vi "S4GUI.vi"(7 "Tab ObsEng":enum32{"Obs", "CCD modes", "Guider", "Eng"}(tab)) -> ()   [LabVIEW 2018] (continued)
        n2655 = call "Write ASEL.vi"("error in (no error)"=w5580, "Opt_Selector.lvclass"=w5582, "Instrument in"=w5591) -> ("error out"=w5542:errorcluster, "Instrument out"=w5558:refnum<class "Instrument.lvclass">)  [unwired: 7 in]
        n2656 = call "Read CALW.vi"("error in (no error)"=w5542, "Instrument in"=w5558) -> ("error out"=w5575:errorcluster, "Opt_Selector.lvclass"=w5576:refnum<class "Opt_Selector.lvclass">, "Instrument out"=w5557:refnum<class "Instrument.lvclass">)  [unwired: 7 in]
        n2657 = call-dynamic "Read State Machine.vi"("error in (no error)"=w5575, "Device in"=w5576) -> ("error out"=w5572:errorcluster, "State Machine.lvclass"=w5570:refnum<class "State Machine.lvclass">, "Device out"=w5578:refnum<class "Opt_Selector.lvclass">)  [unwired: 7 in]
        n2658 = call "Next State.vi"("error in (no error)"=w5572, "New_State"=1, "State Machine in"=w5570) -> ("error out"=w5573:errorcluster, "State Machine out"=w5574:refnum<class "State Machine.lvclass">)  [unwired: 7 in]
        n2659 = call-dynamic "Write State Machine.vi"("error in (no error)"=w5573, "State Machine.lvclass"=w5574, "Device in"=w5578) -> ("error out"=w5579:errorcluster, "Device out"=w5577:refnum<class "Opt_Selector.lvclass">)  [unwired: 7 in]
        n2660 = call "Write CALW.vi"("error in (no error)"=w5579, "Opt_Selector.lvclass"=w5577, "Instrument in"=w5557) -> ("error out"=w5541:errorcluster, "Instrument out"=w5556:refnum<class "Instrument.lvclass">)  [unwired: 7 in]
        n2661 = call "Read WPSEL.vi"("error in (no error)"=w5541, "Instrument in"=w5556) -> ("error out"=w5564:errorcluster, "Opt_Selector.lvclass"=w5563:refnum<class "Opt_Selector.lvclass">, "Instrument out"=w5555:refnum<class "Instrument.lvclass">)  [unwired: 7 in]
        n2662 = call-dynamic "Read State Machine.vi"("error in (no error)"=w5564, "Device in"=w5563) -> ("error out"=w5567:errorcluster, "State Machine.lvclass"=w5569:refnum<class "State Machine.lvclass">, "Device out"=w5561:refnum<class "Opt_Selector.lvclass">)  [unwired: 7 in]
        n2663 = call "Next State.vi"("error in (no error)"=w5567, "New_State"=1, "State Machine in"=w5569) -> ("error out"=w5566:errorcluster, "State Machine out"=w5565:refnum<class "State Machine.lvclass">)  [unwired: 7 in]
        n2664 = call-dynamic "Write State Machine.vi"("error in (no error)"=w5566, "State Machine.lvclass"=w5565, "Device in"=w5561) -> ("error out"=w5560:errorcluster, "Device out"=w5562:refnum<class "Opt_Selector.lvclass">)  [unwired: 7 in]
        n2665 = call "Write WPSEL.vi"("error in (no error)"=w5560, "Opt_Selector.lvclass"=w5562, "Instrument in"=w5555) -> ("error out"=w5540:errorcluster, "Instrument out"=w5544:refnum<class "Instrument.lvclass">)  [unwired: 7 in]
        n2666 = call "Read WPROT.vi"("error in (no error)"=w5540, "Instrument in"=w5544) -> ("error out"=w5550:errorcluster, "Opt_Selector.lvclass"=w5551:refnum<class "Opt_Selector.lvclass">, "Instrument out"=w5543:refnum<class "Instrument.lvclass">)  [unwired: 7 in]
        n2667 = call-dynamic "Read State Machine.vi"("error in (no error)"=w5550, "Device in"=w5551) -> ("error out"=w5547:errorcluster, "State Machine.lvclass"=w5545:refnum<class "State Machine.lvclass">, "Device out"=w5553:refnum<class "Opt_Selector.lvclass">)  [unwired: 7 in]
        n2668 = call "Next State.vi"("error in (no error)"=w5547, "New_State"=1, "State Machine in"=w5545) -> ("error out"=w5548:errorcluster, "State Machine out"=w5549:refnum<class "State Machine.lvclass">)  [unwired: 7 in]
        n2669 = call-dynamic "Write State Machine.vi"("error in (no error)"=w5548, "State Machine.lvclass"=w5549, "Device in"=w5553) -> ("error out"=w5554:errorcluster, "Device out"=w5552:refnum<class "Opt_Selector.lvclass">)  [unwired: 7 in]
        n2670 = call "Write WPROT.vi"("error in (no error)"=w5554, "Opt_Selector.lvclass"=w5552, "Instrument in"=w5543) -> ("error out"=w5516:errorcluster, "Instrument out"=w5517:refnum<class "Instrument.lvclass">)  [unwired: 7 in]
        n2671 = call "Read GMIR.vi"("error in (no error)"=w5516, "Instrument in"=w5517) -> ("error out"=w5535:errorcluster, "Opt_Continuous.lvclass"=w5536:refnum<class "Opt_Continuous.lvclass">, "Instrument out"=w5529:refnum<class "Instrument.lvclass">)  [unwired: 7 in]
        n2672 = call-dynamic "Read State Machine.vi"("error in (no error)"=w5535, "Device in"=w5536) -> ("error out"=w5532:errorcluster, "State Machine.lvclass"=w5530:refnum<class "State Machine.lvclass">, "Device out"=w5538:refnum<class "Opt_Continuous.lvclass">)  [unwired: 7 in]
        n2673 = call "Next State.vi"("error in (no error)"=w5532, "New_State"=1, "State Machine in"=w5530) -> ("error out"=w5533:errorcluster, "State Machine out"=w5534:refnum<class "State Machine.lvclass">)  [unwired: 7 in]
        n2674 = call-dynamic "Write State Machine.vi"("error in (no error)"=w5533, "State Machine.lvclass"=w5534, "Device in"=w5538) -> ("error out"=w5539:errorcluster, "Device out"=w5537:refnum<class "Opt_Continuous.lvclass">)  [unwired: 7 in]
        n2675 = call "Write GMIR.vi"("error in (no error)"=w5539, "Opt_Continuous.lvclass"=w5537, "Instrument in"=w5529) -> ("error out"=w5514:errorcluster, "Instrument out"=w5515:refnum<class "Instrument.lvclass">)  [unwired: 7 in]
        n2676 = call "Read GFOC.vi"("error in (no error)"=w5514, "Instrument in"=w5515) -> ("error out"=w5524:errorcluster, "Opt_Continuous.lvclass"=w5525:refnum<class "Opt_Continuous.lvclass">, "Instrument out"=w5518:refnum<class "Instrument.lvclass">)  [unwired: 7 in]
        n2677 = call-dynamic "Read State Machine.vi"("error in (no error)"=w5524, "Device in"=w5525) -> ("error out"=w5521:errorcluster, "State Machine.lvclass"=w5519:refnum<class "State Machine.lvclass">, "Device out"=w5527:refnum<class "Opt_Continuous.lvclass">)  [unwired: 7 in]
        n2678 = call "Next State.vi"("error in (no error)"=w5521, "New_State"=1, "State Machine in"=w5519) -> ("error out"=w5522:errorcluster, "State Machine out"=w5523:refnum<class "State Machine.lvclass">)  [unwired: 7 in]
        n2679 = call-dynamic "Write State Machine.vi"("error in (no error)"=w5522, "State Machine.lvclass"=w5523, "Device in"=w5527) -> ("error out"=w5528:errorcluster, "Device out"=w5526:refnum<class "Opt_Continuous.lvclass">)  [unwired: 7 in]
        n2680 = call "Write GFOC.vi"("error in (no error)"=w5528, "Opt_Continuous.lvclass"=w5526, "Instrument in"=w5518) -> ("error out"=w5510:errorcluster, "Instrument out"=w5511:refnum<class "Instrument.lvclass">)  [unwired: 7 in]
        n2681 = call "Write Instrument.lvclass.vi"("error in (no error)"=w5510, "Instrument.lvclass"=w5511, "S4ACS_GUI in"=w5590) -> ("error out"=w5509:errorcluster, "S4ACS_GUI out"=w5508:refnum<class "S4GUI.lvclass">)  [unwired: 7 in]
      }
      event "Tab Acq Type": Value Change {
        # "Tab for choosing ACQUISITION MODE: Object, Test, Dflat, Sflat, Dark, Zero, Focus"
        n2682 = event-data() -> ("NewVal"=w5631:T1)  [unwired: 1 in]
        n2683 = case shown="\"TEST\"" w5631 {
          tunnel: ["OBJECT" "OBJECT" "FLAT" "FLAT" "DARK" "ZERO" "FOCUS"] -> w5608
          tunnel: [w5700 w5705 w5713 w5718 w5723 w5728 w5733] -> w5607
          tunnel: [w5701 w5706 w5712 w5717 w5722 w5727 w5732] -> w5630
          tunnel: [w5702 w5707 w5711 w5716 w5721 w5726 w5731] -> w5604
          tunnel: [u32 0 u32 1 u32 2 u32 3 u32 4 u32 5 u32 6] -> w5593
          frame "OBJECT", Default {
            n2684 = local read "Object_obj"() -> (w5700:string)
            n2685 = local read "OBJECT Comments"() -> (w5702:string)
            n2686 = local read "object suffix"() -> (w5701:string)
          }
          frame "TEST" {
            n2687 = local read "TEST Comments"() -> (w5707:string)
            n2688 = local read "Object_test"() -> (w5705:string)
            n2689 = local read "test suffix"() -> (w5706:string)
          }
          frame "DFLAT" {
            n2690 = local read "DFLAT Comments"() -> (w5711:string)
            n2691 = local read "Object_dflat"() -> (w5713:string)
            n2692 = local read "dflat suffix"() -> (w5712:string)
          }
          frame "SFLAT" {
            n2693 = local read "SFLAT Comments"() -> (w5716:string)
            n2694 = local read "Object_sflat"() -> (w5718:string)
            n2695 = local read "sflat suffix"() -> (w5717:string)
          }
          frame "DARK" {
            n2696 = local read "Object_dark"() -> (w5723:string)
            n2697 = local read "dark suffix"() -> (w5722:string)
            n2698 = local read "DARK Comments"() -> (w5721:string)
          }
          frame "ZERO" {
            n2699 = local read "ZERO Comments"() -> (w5726:string)
            n2700 = local read "Object_zero"() -> (w5728:string)
            n2701 = local read "zero suffix"() -> (w5727:string)
          }
          frame "FOCUS" {
            n2702 = local read "FOCUS Comments"() -> (w5731:string)
            n2703 = local read "Object_focus"() -> (w5733:string)
            n2704 = local read "focus suffix"() -> (w5732:string)
          }
        }
        n2705 = local read "Observer"() -> (w5629:string)
        n2706 = call-dynamic "Write ExpMode.vi"("error in (no error)"=w5632, "ExpMode"=w5631, "S4GUI in"=w5633) -> ("error out"=w5625:errorcluster, "S4GUI out"=w5624:refnum<class "S4GUI.lvclass">)  [unwired: 7 in]
        n2707 = Concatenate Strings("ACQ TAB SELECTED:" ("User Event"), w5608) -> (w5626:string)
        n2708 = call-dynamic "Write User Event.vi"("error in (no error)"=w5625, "User Event"=w5626, "S4GUI in"=w5624) -> ("error out"=w5598:errorcluster, "S4GUI out"=w5599:refnum<class "S4GUI.lvclass">)  [unwired: 7 in]
        n2709 = call-dynamic "Write TabAcqType index.vi"("error in (no error)"=w5598, "TabAcqType index"=w5593, "S4GUI in"=w5599) -> ("error out"=w5597:errorcluster, "S4GUI out"=w5595:refnum<class "S4GUI.lvclass">)  [unwired: 7 in]
        n2710 = call-dynamic "Save TabAcqType index.vi"("error in (no error)"=w5597, "S4GUI in"=w5595) -> ("error out"=w5596:errorcluster, "S4GUI out"=w5594:refnum<class "S4GUI.lvclass">)  [unwired: 8 in]
        n2711 = call-dynamic "Read Publisher.lvclass.vi"("error in (no error)"=w5596, "S4GUI in"=w5594) -> ("error out"=w5622:errorcluster, "Publisher.lvclass"=w5618:refnum<class "Publisher.lvclass">, "S4GUI out"=w5623:refnum<class "S4GUI.lvclass">)  [unwired: 7 in]
        n2712 = call-dynamic "Write object.vi"("error in (no error)"=w5622, "object"=w5607, "Publisher in"=w5618) -> ("error out"=w5621:errorcluster, "Publisher out"=w5617:refnum<class "Publisher.lvclass">)  [unwired: 7 in]
        n2713 = call-dynamic "Write obstype.vi"("error in (no error)"=w5621, "obstype"=w5608, "Publisher in"=w5617) -> ("error out"=w5620:errorcluster, "Publisher out"=w5616:refnum<class "Publisher.lvclass">)  [unwired: 7 in]
        n2714 = call-dynamic "Write observer.vi"("error in (no error)"=w5620, "observer"=w5606, "Publisher in"=w5616) -> ("error out"=w5619:errorcluster, "Publisher out"=w5615:refnum<class "Publisher.lvclass">)  [unwired: 7 in]
        n2715 = call-dynamic "Write projid.vi"("error in (no error)"=w5619, "projid"=w5605, "Publisher in"=w5615) -> ("error out"=w5612:errorcluster, "Publisher out"=w5611:refnum<class "Publisher.lvclass">)  [unwired: 7 in]
        n2716 = call-dynamic "Write comments.vi"("error in (no error)"=w5612, "comments"=w5604, "Publisher in"=w5611) -> ("error out"=w5614:errorcluster, "Publisher out"=w5613:refnum<class "Publisher.lvclass">)  [unwired: 7 in]
        n2717 = call-dynamic "Write Publisher.lvclass.vi"("error in (no error)"=w5614, "Publisher.lvclass"=w5613, "S4GUI in"=w5623) -> ("error out"=w5610:errorcluster, "S4GUI out"=w5609:refnum<class "S4GUI.lvclass">)  [unwired: 7 in]
        n2718 = call-dynamic "Read AcquisitionA.vi"("error in (no error)"=w5610, "S4ACS_GUI in"=w5609) -> ("error out"=w5640:errorcluster, "Acquisition.lvclass"=w5641:refnum<class "Acquisition.lvclass">, "S4ACS_GUI out"=w5660:refnum<class "S4GUI.lvclass">)  [unwired: 7 in]
        n2719 = call-dynamic "Read AcquisitionC.vi"("error in (no error)"=w5596, "S4ACS_GUI in"=w5594) -> ("error out"=w5636:errorcluster, "Acquisition.lvclass"=w5637:refnum<class "Acquisition.lvclass">)  [unwired: 7 in, 1 out]
        n2720 = call "Read AcquisitionB.vi"("error in (no error)"=w5596, "S4ACS_GUI in"=w5594) -> ("error out"=w5638:errorcluster, "Acquisition.lvclass"=w5639:refnum<class "Acquisition.lvclass">)  [unwired: 7 in, 1 out]
        n2721 = call-dynamic "Read AcquisitionD.vi"("error in (no error)"=w5596, "S4ACS_GUI in"=w5594) -> ("error out"=w5634:errorcluster, "Acquisition.lvclass"=w5635:refnum<class "Acquisition.lvclass">)  [unwired: 7 in, 1 out]
        n2722 = To Lower Case(string=w5630) -> (all lower case string=w5628:string)
        n2723 = case shown="\"OBJECT\", Default" w5631 {
          tunnel: [w5968 w6337 w6770] -> w5659
          tunnel: [w5967 w6336 w6769] -> w5658
          tunnel: [w5966 w6335 w6768] -> w5656
          tunnel: [w5965 w6334 w6767] -> w5655
          tunnel: [w5964 w6333 w6766] -> w5645
          tunnel: [w5963 w6332 w6765] -> w5644
          tunnel: [w5962 w6331 w6764] -> w5643
          tunnel: [w5961 w6330 w6763] -> w5642
          tunnel: w5641 -> [w5960 w6329 w6762]
          tunnel: w5640 -> [w5959 w6328 w6761]
          tunnel: w5639 -> [w5949 w6319 w6752]
          tunnel: w5638 -> [w5948 w6318 w6751]
          tunnel: w5637 -> [w5947 w6317 w6750]
          tunnel: w5636 -> [w5946 w6316 w6749]
          tunnel: w5635 -> [w5945 w6315 w6748]
          tunnel: w5634 -> [w5944 w6314 w6747]
          tunnel: w5607 -> [w5941 w6313 w6746]
          tunnel: w5604 -> [w5942 w6312 w6745]
          tunnel: w5629 -> [w5943 w6311 w6744]
          tunnel: w5628 -> [w5940 w6310 w6743]
          tunnel: w5608 -> [w5939 w6309 w6742]
          frame "ZERO" {
            w5958 = 1e-05 ("Exptime ch1")
            # "nome do arquivo .cfg"
            # "seção no arquivo .cfg"
            # "nome do arquivo .cfg"
            # "seção no arquivo .cfg"
            # "nome do arquivo .cfg"
            # "seção no arquivo .cfg"
            # "nome do arquivo .cfg"
            # "seção no arquivo .cfg"
            # "ZERO: EXPTIME=1E-5 (mandatory), shutter automatically closed, save current FRAME_TRANSFER (prev_FT) and reset FRAME_TRANSFER."
            n2724 = call "Read connection.vi"("error in (no error)"=w5946, "Server in"=w5947) -> ("error out"=w5952:errorcluster, "connection"=w5786:bool, "Server out"=w5953:refnum<class "Acquisition.lvclass">)  [unwired: 7 in]
            n2725 = call "Read connection.vi"("error in (no error)"=w5948, "Server in"=w5949) -> ("error out"=w5954:errorcluster, "connection"=w5837:bool, "Server out"=w5955:refnum<class "Acquisition.lvclass">)  [unwired: 7 in]
            n2726 = call "Read connection.vi"("error in (no error)"=w5959, "Server in"=w5960) -> ("error out"=w5956:errorcluster, "connection"=w5888:bool, "Server out"=w5957:refnum<class "Acquisition.lvclass">)  [unwired: 7 in]
            n2727 = call "Read connection.vi"("error in (no error)"=w5944, "Server in"=w5945) -> ("error out"=w5950:errorcluster, "connection"=w5735:bool, "Server out"=w5951:refnum<class "Acquisition.lvclass">)  [unwired: 7 in]
            n2728 = call-dynamic "Read Channel.vi"("error in (no error)"=w5954, "Acquisition in"=w5955) -> ("error out"=w5875:errorcluster, "Channel.lvclass"=w5874:refnum<class "Channel.lvclass">, "Acquisition out"=w5873:refnum<class "Acquisition.lvclass">)  [unwired: 7 in]
            n2729 = call-dynamic "Read Channel.vi"("error in (no error)"=w5950, "Acquisition in"=w5951) -> ("error out"=w5783:errorcluster, "Channel.lvclass"=w5784:refnum<class "Channel.lvclass">, "Acquisition out"=w5785:refnum<class "Acquisition.lvclass">)  [unwired: 7 in]
            n2730 = call-dynamic "Read Channel.vi"("error in (no error)"=w5952, "Acquisition in"=w5953) -> ("error out"=w5824:errorcluster, "Channel.lvclass"=w5823:refnum<class "Channel.lvclass">, "Acquisition out"=w5822:refnum<class "Acquisition.lvclass">)  [unwired: 7 in]
            n2731 = call-dynamic "Read Channel.vi"("error in (no error)"=w5956, "Acquisition in"=w5957) -> ("error out"=w5936:errorcluster, "Channel.lvclass"=w5937:refnum<class "Channel.lvclass">, "Acquisition out"=w5938:refnum<class "Acquisition.lvclass">)  [unwired: 7 in]
            n2732 = call-dynamic "Read Interface.vi"("error in (no error)"=w5783, "Channel in"=w5784) -> ("error out"=w5749:errorcluster, "Interface.lvclass"=w5748:refnum<class "Interface.lvclass">, "Channel out"=w5745:refnum<class "Channel.lvclass">)  [unwired: 7 in]
            n2733 = call-dynamic "Read Interface.vi"("error in (no error)"=w5875, "Channel in"=w5874) -> ("error out"=w5849:errorcluster, "Interface.lvclass"=w5850:refnum<class "Interface.lvclass">, "Channel out"=w5844:refnum<class "Channel.lvclass">)  [unwired: 7 in]
            n2734 = call-dynamic "Read Interface.vi"("error in (no error)"=w5824, "Channel in"=w5823) -> ("error out"=w5798:errorcluster, "Interface.lvclass"=w5799:refnum<class "Interface.lvclass">, "Channel out"=w5796:refnum<class "Channel.lvclass">)  [unwired: 7 in]
            n2735 = call-dynamic "Read Interface.vi"("error in (no error)"=w5936, "Channel in"=w5937) -> ("error out"=w5905:errorcluster, "Interface.lvclass"=w5906:refnum<class "Interface.lvclass">, "Channel out"=w5899:refnum<class "Channel.lvclass">)  [unwired: 7 in]
            n2736 = call-dynamic "Write restoreExpTime.vi"("error in (no error)"=w5749, "restoreExpTime"=TRUE, "Interface in"=w5748) -> ("error out"=w5742:errorcluster, "Interface out"=w5747:refnum<class "Interface.lvclass">)  [unwired: 7 in]
            n2737 = call-dynamic "Write restoreExpTime.vi"("error in (no error)"=w5849, "restoreExpTime"=TRUE, "Interface in"=w5850) -> ("error out"=w5846:errorcluster, "Interface out"=w5848:refnum<class "Interface.lvclass">)  [unwired: 7 in]
            n2738 = call-dynamic "Write restoreExpTime.vi"("error in (no error)"=w5798, "restoreExpTime"=TRUE, "Interface in"=w5799) -> ("error out"=w5791:errorcluster, "Interface out"=w5797:refnum<class "Interface.lvclass">)  [unwired: 7 in]
            n2739 = call-dynamic "Write restoreExpTime.vi"("error in (no error)"=w5905, "restoreExpTime"=TRUE, "Interface in"=w5906) -> ("error out"=w5895:errorcluster, "Interface out"=w5896:refnum<class "Interface.lvclass">)  [unwired: 7 in]
            n2740 = property on="Exptime ch1" class="DigNum (strict)"("Value"=w5958) -> ()  [unwired: 2 in, 2 out]
            n2741 = call-dynamic "Read target cluster.vi"("error in (no error)"=w5846, "Channel in"=w5844) -> ("error out"=w5845:errorcluster, "target cluster"=w5847:T31, "Channel out"=w5840:refnum<class "Channel.lvclass">)  [unwired: 7 in]
            n2742 = stacked-sequence {
              tunnel: [_ w6060] -> w5843
              tunnel: w5847 -> [_ w6059]
              tunnel: w5847 -> [w6057 _]
              tunnel: [w6056 _] -> w5852
              frame #0 {
                n2743 = Unbundle By Name(w6057) -> ("FRAME_TRANSFER"=w6056:bool)
              }
              frame #1 {
                # "closed"
                n2744 = Bundle By Name(cluster=w6059, "SHUTTER_MODE"=u8 2, "FRAME_TRANSFER"=FALSE) -> (w6060:T31)
              }
            }
            n2745 = call-dynamic "Read target cluster.vi"("error in (no error)"=w5742, "Channel in"=w5745) -> ("error out"=w5741:errorcluster, "target cluster"=w5743:T31, "Channel out"=w5744:refnum<class "Channel.lvclass">)  [unwired: 7 in]
            n2746 = stacked-sequence {
              tunnel: w5743 -> [_ w5999]
              tunnel: [_ w5998] -> w5739
              tunnel: w5743 -> [w5995 _]
              tunnel: [w5994 _] -> w5751
              frame #0 {
                n2747 = Unbundle By Name(w5995) -> ("FRAME_TRANSFER"=w5994:bool)
              }
              frame #1 {
                # "closed"
                n2748 = Bundle By Name(cluster=w5999, "SHUTTER_MODE"=u8 2, "FRAME_TRANSFER"=FALSE) -> (w5998:T31)
              }
            }
            n2749 = call-dynamic "Read target cluster.vi"("error in (no error)"=w5791, "Channel in"=w5796) -> ("error out"=w5790:errorcluster, "target cluster"=w5792:T31, "Channel out"=w5788:refnum<class "Channel.lvclass">)  [unwired: 7 in]
            n2750 = stacked-sequence {
              tunnel: [_ w6029] -> w5794
              tunnel: w5792 -> [_ w6028]
              tunnel: w5792 -> [w6026 _]
              tunnel: [w6025 _] -> w5801
              frame #0 {
                n2751 = Unbundle By Name(w6026) -> ("FRAME_TRANSFER"=w6025:bool)
              }
              frame #1 {
                # "closed"
                n2752 = Bundle By Name(cluster=w6028, "SHUTTER_MODE"=u8 2, "FRAME_TRANSFER"=FALSE) -> (w6029:T31)
              }
            }
            n2753 = property on="Exptime ch2" class="DigNum (strict)"("Value"=w5958) -> ()  [unwired: 2 in, 2 out]
            n2754 = call-dynamic "Read target cluster.vi"("error in (no error)"=w5895, "Channel in"=w5899) -> ("error out"=w5894:errorcluster, "target cluster"=w5897:T31, "Channel out"=w5898:refnum<class "Channel.lvclass">)  [unwired: 7 in]
            n2755 = stacked-sequence {
              tunnel: [_ w6092] -> w5903
              tunnel: w5897 -> [_ w6089]
              tunnel: w5897 -> [w6088 _]
              tunnel: [w6087 _] -> w5907
              frame #0 {
                n2756 = Unbundle By Name(w6088) -> ("FRAME_TRANSFER"=w6087:bool)
              }
              frame #1 {
                # "closed"
                n2757 = Bundle By Name(cluster=w6089, "SHUTTER_MODE"=u8 2, "FRAME_TRANSFER"=FALSE) -> (w6092:T31)
              }
            }
            n2758 = call-dynamic "Write PREV_FT.vi"("error in (no error)"=w5845, "PREV_FT"=w5852, "Interface in"=w5848) -> ("error out"=w5842:errorcluster, "Interface out"=w5838:refnum<class "Interface.lvclass">)  [unwired: 7 in]
            n2759 = call-dynamic "Write PREV_FT.vi"("error in (no error)"=w5741, "PREV_FT"=w5751, "Interface in"=w5747) -> ("error out"=w5740:errorcluster, "Interface out"=w5746:refnum<class "Interface.lvclass">)  [unwired: 7 in]
            n2760 = call-dynamic "Write PREV_FT.vi"("error in (no error)"=w5790, "PREV_FT"=w5801, "Interface in"=w5797) -> ("error out"=w5793:errorcluster, "Interface out"=w5795:refnum<class "Interface.lvclass">)  [unwired: 7 in]
            n2761 = property on="Exptime ch3" class="DigNum (strict)"("Value"=w5958) -> ()  [unwired: 2 in, 2 out]
            n2762 = call-dynamic "Write PREV_FT.vi"("error in (no error)"=w5894, "PREV_FT"=w5907, "Interface in"=w5896) -> ("error out"=w5900:errorcluster, "Interface out"=w5893:refnum<class "Interface.lvclass">)  [unwired: 7 in]
            n2763 = call-dynamic "Write target cluster.vi"("error in (no error)"=w5842, "target cluster"=w5843, "Channel in"=w5840) -> ("error out"=w5841:errorcluster, "Channel out"=w5839:refnum<class "Channel.lvclass">)  [unwired: 7 in]
            n2764 = call-dynamic "Write target cluster.vi"("error in (no error)"=w5740, "target cluster"=w5739, "Channel in"=w5744) -> ("error out"=w5738:errorcluster, "Channel out"=w5737:refnum<class "Channel.lvclass">)  [unwired: 7 in]
            n2765 = call-dynamic "Write target cluster.vi"("error in (no error)"=w5793, "target cluster"=w5794, "Channel in"=w5788) -> ("error out"=w5789:errorcluster, "Channel out"=w5787:refnum<class "Channel.lvclass">)  [unwired: 7 in]
            n2766 = call-dynamic "Write target cluster.vi"("error in (no error)"=w5900, "target cluster"=w5903, "Channel in"=w5898) -> ("error out"=w5902:errorcluster, "Channel out"=w5901:refnum<class "Channel.lvclass">)  [unwired: 7 in]
            n2767 = Flatten To String(anything=w5843, error in (no error)=w5841) -> (data string=w5876:string, error out=w5877:errorcluster)  [unwired: 2 in, 1 out]
            n2768 = Flatten To String(anything=w5739, error in (no error)=w5738) -> (data string=w5782:string, error out=w5781:errorcluster)  [unwired: 2 in, 1 out]
            n2769 = Flatten To String(anything=w5794, error in (no error)=w5789) -> (data string=w5825:string, error out=w5826:errorcluster)  [unwired: 2 in, 1 out]
            n2770 = Flatten To String(anything=w5903, error in (no error)=w5902) -> (data string=w5935:string, error out=w5934:errorcluster)  [unwired: 2 in, 1 out]
            n2771 = property on="Exptime ch4" class="DigNum (strict)"("Value"=w5958) -> ()  [unwired: 2 in, 2 out]
            n2772 = call "Write flatted cluster.vi"("error in (no error)"=w5877, "flatted cluster"=w5876, "Interface in"=w5838) -> ("error out"=w5879:errorcluster, "Interface out"=w5878:refnum<class "Interface.lvclass">)  [unwired: 7 in]
            n2773 = call "Write flatted cluster.vi"("error in (no error)"=w5781, "flatted cluster"=w5782, "Interface in"=w5746) -> ("error out"=w5779:errorcluster, "Interface out"=w5780:refnum<class "Interface.lvclass">)  [unwired: 7 in]
            n2774 = call "Write flatted cluster.vi"("error in (no error)"=w5826, "flatted cluster"=w5825, "Interface in"=w5795) -> ("error out"=w5828:errorcluster, "Interface out"=w5827:refnum<class "Interface.lvclass">)  [unwired: 7 in]
            n2775 = call "Write flatted cluster.vi"("error in (no error)"=w5934, "flatted cluster"=w5935, "Interface in"=w5893) -> ("error out"=w5932:errorcluster, "Interface out"=w5933:refnum<class "Interface.lvclass">)  [unwired: 7 in]
            n2776 = call-dynamic "Write Interface.vi"("error in (no error)"=w5879, "Interface.lvclass"=w5878, "Channel in"=w5839) -> ("error out"=w5881:errorcluster, "Channel out"=w5882:refnum<class "Channel.lvclass">)  [unwired: 7 in]
            n2777 = call-dynamic "Write Interface.vi"("error in (no error)"=w5779, "Interface.lvclass"=w5780, "Channel in"=w5737) -> ("error out"=w5777:errorcluster, "Channel out"=w5776:refnum<class "Channel.lvclass">)  [unwired: 7 in]
            n2778 = call-dynamic "Write Interface.vi"("error in (no error)"=w5828, "Interface.lvclass"=w5827, "Channel in"=w5787) -> ("error out"=w5830:errorcluster, "Channel out"=w5831:refnum<class "Channel.lvclass">)  [unwired: 7 in]
            n2779 = call-dynamic "Write Interface.vi"("error in (no error)"=w5932, "Interface.lvclass"=w5933, "Channel in"=w5901) -> ("error out"=w5930:errorcluster, "Channel out"=w5929:refnum<class "Channel.lvclass">)  [unwired: 7 in]
            n2780 = call "Write section_name.vi"("error in (no error)"=w5881, "section_name"="CCD_ACS2", "Channel in"=w5882) -> ("error out"=w5880:errorcluster, "Channel out"=w5885:refnum<class "Channel.lvclass">)  [unwired: 7 in]
            n2781 = call "Write section_name.vi"("error in (no error)"=w5777, "section_name"="CCD_ACS4", "Channel in"=w5776) -> ("error out"=w5778:errorcluster, "Channel out"=w5773:refnum<class "Channel.lvclass">)  [unwired: 7 in]
            n2782 = call "Write section_name.vi"("error in (no error)"=w5830, "section_name"="CCD_ACS3", "Channel in"=w5831) -> ("error out"=w5829:errorcluster, "Channel out"=w5834:refnum<class "Channel.lvclass">)  [unwired: 7 in]
            n2783 = call "Write section_name.vi"("error in (no error)"=w5930, "section_name"="CCD_ACS1", "Channel in"=w5929) -> ("error out"=w5931:errorcluster, "Channel out"=w5926:refnum<class "Channel.lvclass">)  [unwired: 7 in]
            n2784 = call-dynamic "save config.vi"("error in (no error)"=w5880, "file config"="lastsaved.cfg", "Channel in"=w5885) -> ("error out"=w5855:errorcluster, "Channel out"=w5856:refnum<class "Channel.lvclass">)  [unwired: 7 in]
            n2785 = call-dynamic "save config.vi"("error in (no error)"=w5778, "file config"="lastsaved.cfg", "Channel in"=w5773) -> ("error out"=w5754:errorcluster, "Channel out"=w5755:refnum<class "Channel.lvclass">)  [unwired: 7 in]
            n2786 = call-dynamic "save config.vi"("error in (no error)"=w5829, "file config"="lastsaved.cfg", "Channel in"=w5834) -> ("error out"=w5803:errorcluster, "Channel out"=w5805:refnum<class "Channel.lvclass">)  [unwired: 7 in]
            n2787 = call-dynamic "save config.vi"("error in (no error)"=w5931, "file config"="lastsaved.cfg", "Channel in"=w5926) -> ("error out"=w5916:errorcluster, "Channel out"=w5917:refnum<class "Channel.lvclass">)  [unwired: 7 in]
            n2788 = local read "Filter2"() -> (w5857:u8)
            n2789 = local read "Filter4"() -> (w5771:u8)
            n2790 = local read "Filter3"() -> (w5821:u8)
            n2791 = local read "Filter1"() -> (w5918:u8)
            n2792 = call-dynamic "Write Filter.vi"("error in (no error)"=w5855, "Filter"=w5857, "Channel in"=w5856) -> ("error out"=w5864:errorcluster, "Channel out"=w5865:refnum<class "Channel.lvclass">)  [unwired: 7 in]
            n2793 = call-dynamic "Write Filter.vi"("error in (no error)"=w5754, "Filter"=w5771, "Channel in"=w5755) -> ("error out"=w5764:errorcluster, "Channel out"=w5763:refnum<class "Channel.lvclass">)  [unwired: 7 in]
            n2794 = call-dynamic "Write Filter.vi"("error in (no error)"=w5803, "Filter"=w5821, "Channel in"=w5805) -> ("error out"=w5814:errorcluster, "Channel out"=w5813:refnum<class "Channel.lvclass">)  [unwired: 7 in]
            n2795 = call-dynamic "Write Filter.vi"("error in (no error)"=w5916, "Filter"=w5918, "Channel in"=w5917) -> ("error out"=w5925:errorcluster, "Channel out"=w5915:refnum<class "Channel.lvclass">)  [unwired: 7 in]
            n2796 = call-dynamic "Read Interface.vi"("error in (no error)"=w5864, "Channel in"=w5865) -> ("error out"=w5862:errorcluster, "Interface.lvclass"=w5867:refnum<class "Interface.lvclass">, "Channel out"=w5866:refnum<class "Channel.lvclass">)  [unwired: 7 in]
            n2797 = call-dynamic "Read Interface.vi"("error in (no error)"=w5764, "Channel in"=w5763) -> ("error out"=w5766:errorcluster, "Interface.lvclass"=w5761:refnum<class "Interface.lvclass">, "Channel out"=w5762:refnum<class "Channel.lvclass">)  [unwired: 7 in]
            n2798 = call-dynamic "Read Interface.vi"("error in (no error)"=w5814, "Channel in"=w5813) -> ("error out"=w5816:errorcluster, "Interface.lvclass"=w5811:refnum<class "Interface.lvclass">, "Channel out"=w5812:refnum<class "Channel.lvclass">)  [unwired: 7 in]
            n2799 = call-dynamic "Read Interface.vi"("error in (no error)"=w5925, "Channel in"=w5915) -> ("error out"=w5923:errorcluster, "Interface.lvclass"=w5914:refnum<class "Interface.lvclass">, "Channel out"=w5908:refnum<class "Channel.lvclass">)  [unwired: 7 in]
            n2800 = call-dynamic "Write Suffix.vi"("error in (no error)"=w5862, "Suffix"=w5940, "Interface in"=w5867) -> ("error out"=w5858:errorcluster, "Interface out"=w5868:refnum<class "Interface.lvclass">)  [unwired: 7 in]
            n2801 = call-dynamic "Write Suffix.vi"("error in (no error)"=w5766, "Suffix"=w5940, "Interface in"=w5761) -> ("error out"=w5770:errorcluster, "Interface out"=w5760:refnum<class "Interface.lvclass">)  [unwired: 7 in]
            n2802 = call-dynamic "Write Suffix.vi"("error in (no error)"=w5816, "Suffix"=w5940, "Interface in"=w5811) -> ("error out"=w5820:errorcluster, "Interface out"=w5810:refnum<class "Interface.lvclass">)  [unwired: 7 in]
            n2803 = call-dynamic "Write Suffix.vi"("error in (no error)"=w5923, "Suffix"=w5940, "Interface in"=w5914) -> ("error out"=w5919:errorcluster, "Interface out"=w5913:refnum<class "Interface.lvclass">)  [unwired: 7 in]
            n2804 = call-dynamic "Write ObsType.vi"("error in (no error)"=w5858, "ObsType"=w5939, "Interface in"=w5868) -> ("error out"=w5859:errorcluster, "Interface out"=w5869:refnum<class "Interface.lvclass">)  [unwired: 7 in]
            n2805 = call-dynamic "Write ObsType.vi"("error in (no error)"=w5770, "ObsType"=w5939, "Interface in"=w5760) -> ("error out"=w5769:errorcluster, "Interface out"=w5759:refnum<class "Interface.lvclass">)  [unwired: 7 in]
            n2806 = call-dynamic "Write ObsType.vi"("error in (no error)"=w5820, "ObsType"=w5939, "Interface in"=w5810) -> ("error out"=w5819:errorcluster, "Interface out"=w5809:refnum<class "Interface.lvclass">)  [unwired: 7 in]
            n2807 = call-dynamic "Write ObsType.vi"("error in (no error)"=w5919, "ObsType"=w5939, "Interface in"=w5913) -> ("error out"=w5920:errorcluster, "Interface out"=w5912:refnum<class "Interface.lvclass">)  [unwired: 7 in]
            n2808 = call-dynamic "Write Object.vi"("error in (no error)"=w5859, "Object"=w5941, "Interface in"=w5869) -> ("error out"=w5860:errorcluster, "Interface out"=w5870:refnum<class "Interface.lvclass">)  [unwired: 7 in]
            n2809 = call-dynamic "Write Object.vi"("error in (no error)"=w5769, "Object"=w5941, "Interface in"=w5759) -> ("error out"=w5768:errorcluster, "Interface out"=w5758:refnum<class "Interface.lvclass">)  [unwired: 7 in]
            n2810 = call-dynamic "Write Object.vi"("error in (no error)"=w5819, "Object"=w5941, "Interface in"=w5809) -> ("error out"=w5818:errorcluster, "Interface out"=w5808:refnum<class "Interface.lvclass">)  [unwired: 7 in]
            n2811 = call-dynamic "Write Object.vi"("error in (no error)"=w5920, "Object"=w5941, "Interface in"=w5912) -> ("error out"=w5921:errorcluster, "Interface out"=w5911:refnum<class "Interface.lvclass">)  [unwired: 7 in]
            n2812 = call-dynamic "Write Comments.vi"("error in (no error)"=w5860, "Comments"=w5942, "Interface in"=w5870) -> ("error out"=w5861:errorcluster, "Interface out"=w5871:refnum<class "Interface.lvclass">)  [unwired: 7 in]
            n2813 = call-dynamic "Write Comments.vi"("error in (no error)"=w5768, "Comments"=w5942, "Interface in"=w5758) -> ("error out"=w5767:errorcluster, "Interface out"=w5757:refnum<class "Interface.lvclass">)  [unwired: 7 in]
            n2814 = call-dynamic "Write Comments.vi"("error in (no error)"=w5818, "Comments"=w5942, "Interface in"=w5808) -> ("error out"=w5817:errorcluster, "Interface out"=w5807:refnum<class "Interface.lvclass">)  [unwired: 7 in]
            n2815 = call-dynamic "Write Comments.vi"("error in (no error)"=w5921, "Comments"=w5942, "Interface in"=w5911) -> ("error out"=w5922:errorcluster, "Interface out"=w5910:refnum<class "Interface.lvclass">)  [unwired: 7 in]
            n2816 = call-dynamic "Write Observer.vi"("error in (no error)"=w5767, "Observer"=w5943, "Interface in"=w5757) -> ("error out"=w5765:errorcluster, "Interface out"=w5756:refnum<class "Interface.lvclass">)  [unwired: 7 in]
            n2817 = call-dynamic "Write Observer.vi"("error in (no error)"=w5817, "Observer"=w5943, "Interface in"=w5807) -> ("error out"=w5815:errorcluster, "Interface out"=w5806:refnum<class "Interface.lvclass">)  [unwired: 7 in]
            n2818 = call-dynamic "Write Observer.vi"("error in (no error)"=w5861, "Observer"=w5943, "Interface in"=w5871) -> ("error out"=w5863:errorcluster, "Interface out"=w5872:refnum<class "Interface.lvclass">)  [unwired: 7 in]
            n2819 = call-dynamic "Write Observer.vi"("error in (no error)"=w5922, "Observer"=w5943, "Interface in"=w5910) -> ("error out"=w5924:errorcluster, "Interface out"=w5909:refnum<class "Interface.lvclass">)  [unwired: 7 in]
            n2820 = call-dynamic "Write Interface.vi"("error in (no error)"=w5765, "Interface.lvclass"=w5756, "Channel in"=w5762) -> ("error out"=w5753:errorcluster, "Channel out"=w5752:refnum<class "Channel.lvclass">)  [unwired: 7 in]
            n2821 = call-dynamic "Write Interface.vi"("error in (no error)"=w5815, "Interface.lvclass"=w5806, "Channel in"=w5812) -> ("error out"=w5802:errorcluster, "Channel out"=w5804:refnum<class "Channel.lvclass">)  [unwired: 7 in]
            n2822 = call-dynamic "Write Interface.vi"("error in (no error)"=w5924, "Interface.lvclass"=w5909, "Channel in"=w5908) -> ("error out"=w5891:errorcluster, "Channel out"=w5892:refnum<class "Channel.lvclass">)  [unwired: 7 in]
            n2823 = call-dynamic "Write Interface.vi"("error in (no error)"=w5863, "Interface.lvclass"=w5872, "Channel in"=w5866) -> ("error out"=w5854:errorcluster, "Channel out"=w5853:refnum<class "Channel.lvclass">)  [unwired: 7 in]
            n2824 = case shown="True" w5888 {
              tunnel: w5892 -> [w6063 w6067]
              tunnel: w5891 -> [w6062 w6066]
              tunnel: [w6063 w6065] -> w5890
              tunnel: [w6062 w6064] -> w5889
              frame False {
              }
              frame True {
                n2825 = call-dynamic "Read State Machine.vi"("error in (no error)"=w6066, "Device in"=w6067) -> ("error out"=w6069:errorcluster, "State Machine.lvclass"=w6072:refnum<class "State Machine.lvclass">, "Device out"=w6084:refnum<class "Channel.lvclass">)  [unwired: 7 in]
                n2826 = call-dynamic "Read ref StatesQueue.vi"("error in (no error)"=w6069, "State Machine in"=w6072) -> ("error out"=w6076:errorcluster, "ref StatesQueue"=w6075:refnum<queue>, "State Machine out"=w6071:refnum<class "State Machine.lvclass">)  [unwired: 7 in]
                n2827 = Flush Queue(queue=w6075, error in (no error)=w6076) -> (queue out=w6077:refnum<queue>, error out=w6081:errorcluster)  [unwired: 1 out]
                n2828 = Enqueue Element(queue=w6077, element=u32 300 ("State"), error in (no error)=w6081) -> (queue out=w6078:refnum<queue>, error out=w6082:errorcluster)  [unwired: 1 in, 1 out]
                n2829 = Enqueue Element(queue=w6078, element=u32 60 ("State"), error in (no error)=w6082) -> (queue out=w6079:refnum<queue>, error out=w6080:errorcluster)  [unwired: 1 in, 1 out]
                n2830 = call-dynamic "Write ref StatesQueue.vi"("error in (no error)"=w6080, "ref StatesQueue"=w6079, "State Machine in"=w6071) -> ("error out"=w6068:errorcluster, "State Machine out"=w6070:refnum<class "State Machine.lvclass">)  [unwired: 7 in]
                n2831 = call-dynamic "Write State.vi"("error in (no error)"=w6068, "State"=0, "State Machine in"=w6070) -> ("error out"=w6086:errorcluster, "State Machine out"=w6083:refnum<class "State Machine.lvclass">)  [unwired: 7 in]
                n2832 = call-dynamic "Write State Machine.vi"("error in (no error)"=w6086, "State Machine.lvclass"=w6083, "Device in"=w6084) -> ("error out"=w6064:errorcluster, "Device out"=w6065:refnum<class "Channel.lvclass">)  [unwired: 7 in]
              }
            }
            n2833 = case shown="True" w5837 {
              tunnel: [w6031 w6055] -> w5887
              tunnel: [w6032 w6054] -> w5886
              tunnel: w5854 -> [w6031 w6049]
              tunnel: w5853 -> [w6032 w6048]
              frame False {
              }
              frame True {
                n2834 = call-dynamic "Read State Machine.vi"("error in (no error)"=w6049, "Device in"=w6048) -> ("error out"=w6034:errorcluster, "State Machine.lvclass"=w6036:refnum<class "State Machine.lvclass">, "Device out"=w6052:refnum<class "Channel.lvclass">)  [unwired: 7 in]
                n2835 = call-dynamic "Read ref StatesQueue.vi"("error in (no error)"=w6034, "State Machine in"=w6036) -> ("error out"=w6041:errorcluster, "ref StatesQueue"=w6040:refnum<queue>, "State Machine out"=w6037:refnum<class "State Machine.lvclass">)  [unwired: 7 in]
                n2836 = Flush Queue(queue=w6040, error in (no error)=w6041) -> (queue out=w6042:refnum<queue>, error out=w6046:errorcluster)  [unwired: 1 out]
                n2837 = Enqueue Element(queue=w6042, element=u32 300 ("State"), error in (no error)=w6046) -> (queue out=w6043:refnum<queue>, error out=w6047:errorcluster)  [unwired: 1 in, 1 out]
                n2838 = Enqueue Element(queue=w6043, element=u32 60 ("State"), error in (no error)=w6047) -> (queue out=w6044:refnum<queue>, error out=w6045:errorcluster)  [unwired: 1 in, 1 out]
                n2839 = call-dynamic "Write ref StatesQueue.vi"("error in (no error)"=w6045, "ref StatesQueue"=w6044, "State Machine in"=w6037) -> ("error out"=w6033:errorcluster, "State Machine out"=w6035:refnum<class "State Machine.lvclass">)  [unwired: 7 in]
                n2840 = call-dynamic "Write State.vi"("error in (no error)"=w6033, "State"=0, "State Machine in"=w6035) -> ("error out"=w6050:errorcluster, "State Machine out"=w6053:refnum<class "State Machine.lvclass">)  [unwired: 7 in]
                n2841 = call-dynamic "Write State Machine.vi"("error in (no error)"=w6050, "State Machine.lvclass"=w6053, "Device in"=w6052) -> ("error out"=w6055:errorcluster, "Device out"=w6054:refnum<class "Channel.lvclass">)  [unwired: 7 in]
              }
            }
            n2842 = case shown="True" w5786 {
              tunnel: [w6001 w6024] -> w5836
              tunnel: [w6000 w6023] -> w5835
              tunnel: w5804 -> [w6000 w6018]
              tunnel: w5802 -> [w6001 w6017]
              frame False {
              }
              frame True {
                n2843 = call-dynamic "Read State Machine.vi"("error in (no error)"=w6017, "Device in"=w6018) -> ("error out"=w6003:errorcluster, "State Machine.lvclass"=w6005:refnum<class "State Machine.lvclass">, "Device out"=w6021:refnum<class "Channel.lvclass">)  [unwired: 7 in]
                n2844 = call-dynamic "Read ref StatesQueue.vi"("error in (no error)"=w6003, "State Machine in"=w6005) -> ("error out"=w6010:errorcluster, "ref StatesQueue"=w6009:refnum<queue>, "State Machine out"=w6006:refnum<class "State Machine.lvclass">)  [unwired: 7 in]
                n2845 = Flush Queue(queue=w6009, error in (no error)=w6010) -> (queue out=w6011:refnum<queue>, error out=w6015:errorcluster)  [unwired: 1 out]
                n2846 = Enqueue Element(queue=w6011, element=u32 300 ("State"), error in (no error)=w6015) -> (queue out=w6012:refnum<queue>, error out=w6016:errorcluster)  [unwired: 1 in, 1 out]
                n2847 = Enqueue Element(queue=w6012, element=u32 60 ("State"), error in (no error)=w6016) -> (queue out=w6013:refnum<queue>, error out=w6014:errorcluster)  [unwired: 1 in, 1 out]
                n2848 = call-dynamic "Write ref StatesQueue.vi"("error in (no error)"=w6014, "ref StatesQueue"=w6013, "State Machine in"=w6006) -> ("error out"=w6002:errorcluster, "State Machine out"=w6004:refnum<class "State Machine.lvclass">)  [unwired: 7 in]
                n2849 = call-dynamic "Write State.vi"("error in (no error)"=w6002, "State"=0, "State Machine in"=w6004) -> ("error out"=w6019:errorcluster, "State Machine out"=w6022:refnum<class "State Machine.lvclass">)  [unwired: 7 in]
                n2850 = call-dynamic "Write State Machine.vi"("error in (no error)"=w6019, "State Machine.lvclass"=w6022, "Device in"=w6021) -> ("error out"=w6024:errorcluster, "Device out"=w6023:refnum<class "Channel.lvclass">)  [unwired: 7 in]
              }
            }
            n2851 = case shown="True" w5735 {
              tunnel: [w5969 w5989] -> w5772
              tunnel: w5753 -> [w5969 w5988]
              tunnel: w5752 -> [w5970 w5987]
              tunnel: [w5970 w5971] -> w5736
              frame False {
              }
              frame True {
                n2852 = call-dynamic "Read State Machine.vi"("error in (no error)"=w5988, "Device in"=w5987) -> ("error out"=w5974:errorcluster, "State Machine.lvclass"=w5975:refnum<class "State Machine.lvclass">, "Device out"=w5991:refnum<class "Channel.lvclass">)  [unwired: 7 in]
                n2853 = call-dynamic "Read ref StatesQueue.vi"("error in (no error)"=w5974, "State Machine in"=w5975) -> ("error out"=w5980:errorcluster, "ref StatesQueue"=w5979:refnum<queue>, "State Machine out"=w5976:refnum<class "State Machine.lvclass">)  [unwired: 7 in]
                n2854 = Flush Queue(queue=w5979, error in (no error)=w5980) -> (queue out=w5981:refnum<queue>, error out=w5985:errorcluster)  [unwired: 1 out]
                n2855 = Enqueue Element(queue=w5981, element=u32 300 ("State"), error in (no error)=w5985) -> (queue out=w5982:refnum<queue>, error out=w5986:errorcluster)  [unwired: 1 in, 1 out]
                n2856 = Enqueue Element(queue=w5982, element=u32 60 ("State"), error in (no error)=w5986) -> (queue out=w5983:refnum<queue>, error out=w5984:errorcluster)  [unwired: 1 in, 1 out]
                n2857 = call-dynamic "Write ref StatesQueue.vi"("error in (no error)"=w5984, "ref StatesQueue"=w5983, "State Machine in"=w5976) -> ("error out"=w5973:errorcluster, "State Machine out"=w5972:refnum<class "State Machine.lvclass">)  [unwired: 7 in]
                n2858 = call-dynamic "Write State.vi"("error in (no error)"=w5973, "State"=0, "State Machine in"=w5972) -> ("error out"=w5993:errorcluster, "State Machine out"=w5990:refnum<class "State Machine.lvclass">)  [unwired: 7 in]
                n2859 = call-dynamic "Write State Machine.vi"("error in (no error)"=w5993, "State Machine.lvclass"=w5990, "Device in"=w5991) -> ("error out"=w5989:errorcluster, "Device out"=w5971:refnum<class "Channel.lvclass">)  [unwired: 7 in]
              }
            }
            n2860 = call-dynamic "Write Channel.vi"("error in (no error)"=w5887, "Channel.lvclass"=w5886, "Acquisition in"=w5873) -> ("error out"=w5965:errorcluster, "Acquisition out"=w5966:refnum<class "Acquisition.lvclass">)  [unwired: 7 in]
            n2861 = call-dynamic "Write Channel.vi"("error in (no error)"=w5889, "Channel.lvclass"=w5890, "Acquisition in"=w5938) -> ("error out"=w5967:errorcluster, "Acquisition out"=w5968:refnum<class "Acquisition.lvclass">)  [unwired: 7 in]
            n2862 = call-dynamic "Write Channel.vi"("error in (no error)"=w5836, "Channel.lvclass"=w5835, "Acquisition in"=w5822) -> ("error out"=w5963:errorcluster, "Acquisition out"=w5964:refnum<class "Acquisition.lvclass">)  [unwired: 7 in]
            n2863 = call-dynamic "Write Channel.vi"("error in (no error)"=w5772, "Channel.lvclass"=w5736, "Acquisition in"=w5785) -> ("error out"=w5961:errorcluster, "Acquisition out"=w5962:refnum<class "Acquisition.lvclass">)  [unwired: 7 in]
          }
          frame "DARK" {
            # "20250918:\nACS corrigido,\nnão precisa restaurar\nExpTime. Causou bug\nquando ExpTime tinha\nvalor default (1E-5s)"
            # "nome do arquivo .cfg"
            # "seção no arquivo .cfg"
            # "closed"
            # "nome do arquivo .cfg"
            # "seção no arquivo .cfg"
            # "closed"
            # "nome do arquivo .cfg"
            # "seção no arquivo .cfg"
            # "closed"
            # "nome do arquivo .cfg"
            # "seção no arquivo .cfg"
            # "closed"
            # "DARK: Shutter automatically closed and restore FRAME_TRANSFER."
            n2864 = call "Read connection.vi"("error in (no error)"=w6314, "Server in"=w6315) -> ("error out"=w6320:errorcluster, "connection"=w6093:bool, "Server out"=w6321:refnum<class "Acquisition.lvclass">)  [unwired: 7 in]
            n2865 = call "Read connection.vi"("error in (no error)"=w6316, "Server in"=w6317) -> ("error out"=w6322:errorcluster, "connection"=w6094:bool, "Server out"=w6323:refnum<class "Acquisition.lvclass">)  [unwired: 7 in]
            n2866 = call "Read connection.vi"("error in (no error)"=w6318, "Server in"=w6319) -> ("error out"=w6324:errorcluster, "connection"=w6095:bool, "Server out"=w6325:refnum<class "Acquisition.lvclass">)  [unwired: 7 in]
            n2867 = call "Read connection.vi"("error in (no error)"=w6328, "Server in"=w6329) -> ("error out"=w6326:errorcluster, "connection"=w6096:bool, "Server out"=w6327:refnum<class "Acquisition.lvclass">)  [unwired: 7 in]
            n2868 = call-dynamic "Read Channel.vi"("error in (no error)"=w6320, "Acquisition in"=w6321) -> ("error out"=w6147:errorcluster, "Channel.lvclass"=w6148:refnum<class "Channel.lvclass">, "Acquisition out"=w6149:refnum<class "Acquisition.lvclass">)  [unwired: 7 in]
            n2869 = call-dynamic "Read Channel.vi"("error in (no error)"=w6322, "Acquisition in"=w6323) -> ("error out"=w6189:errorcluster, "Channel.lvclass"=w6188:refnum<class "Channel.lvclass">, "Acquisition out"=w6187:refnum<class "Acquisition.lvclass">)  [unwired: 7 in]
            n2870 = call-dynamic "Read Channel.vi"("error in (no error)"=w6324, "Acquisition in"=w6325) -> ("error out"=w6242:errorcluster, "Channel.lvclass"=w6241:refnum<class "Channel.lvclass">, "Acquisition out"=w6240:refnum<class "Acquisition.lvclass">)  [unwired: 7 in]
            n2871 = call-dynamic "Read Channel.vi"("error in (no error)"=w6326, "Acquisition in"=w6327) -> ("error out"=w6306:errorcluster, "Channel.lvclass"=w6307:refnum<class "Channel.lvclass">, "Acquisition out"=w6308:refnum<class "Acquisition.lvclass">)  [unwired: 7 in]
            n2872 = call-dynamic "Read Interface.vi"("error in (no error)"=w6147, "Channel in"=w6148) -> ("error out"=w6110:errorcluster, "Interface.lvclass"=w6109:refnum<class "Interface.lvclass">, "Channel out"=w6105:refnum<class "Channel.lvclass">)  [unwired: 7 in]
            n2873 = call-dynamic "Read Interface.vi"("error in (no error)"=w6189, "Channel in"=w6188) -> ("error out"=w6161:errorcluster, "Interface.lvclass"=w6163:refnum<class "Interface.lvclass">, "Channel out"=w6158:refnum<class "Channel.lvclass">)  [unwired: 7 in]
            n2874 = call-dynamic "Read Interface.vi"("error in (no error)"=w6242, "Channel in"=w6241) -> ("error out"=w6216:errorcluster, "Interface.lvclass"=w6215:refnum<class "Interface.lvclass">, "Channel out"=w6211:refnum<class "Channel.lvclass">)  [unwired: 7 in]
            n2875 = call-dynamic "Read Interface.vi"("error in (no error)"=w6306, "Channel in"=w6307) -> ("error out"=w6268:errorcluster, "Interface.lvclass"=w6269:refnum<class "Interface.lvclass">, "Channel out"=w6264:refnum<class "Channel.lvclass">)  [unwired: 7 in]
            n2876 = call-dynamic "Read restoreExpTime.vi"("error in (no error)"=w6110, "Interface in"=w6109) -> ("error out"=w6107:errorcluster, "restoreExpTime"=w6106:bool, "Interface out"=w6108:refnum<class "Interface.lvclass">)  [unwired: 7 in]
            n2877 = call-dynamic "Read restoreExpTime.vi"("error in (no error)"=w6161, "Interface in"=w6163) -> ("error out"=w6160:errorcluster, "restoreExpTime"=w6159:bool, "Interface out"=w6162:refnum<class "Interface.lvclass">)  [unwired: 7 in]
            n2878 = call-dynamic "Read restoreExpTime.vi"("error in (no error)"=w6216, "Interface in"=w6215) -> ("error out"=w6213:errorcluster, "restoreExpTime"=w6212:bool, "Interface out"=w6214:refnum<class "Interface.lvclass">)  [unwired: 7 in]
            n2879 = call-dynamic "Read restoreExpTime.vi"("error in (no error)"=w6268, "Interface in"=w6269) -> ("error out"=w6266:errorcluster, "restoreExpTime"=w6265:bool, "Interface out"=w6267:refnum<class "Interface.lvclass">)  [unwired: 7 in]
            n2880 = case shown="True" w6106 {
              tunnel: w6108 -> [w6475 w6486]
              tunnel: w6107 -> [w6474 w6484]
              tunnel: [w6474 w6477] -> w6112
              tunnel: [w6475 w6476] -> w6111
              frame False {
              }
              frame True {
                n2881 = call-dynamic "Write restoreExpTime.vi"("error in (no error)"=w6484, "restoreExpTime"=FALSE, "Interface in"=w6486) -> ("error out"=w6482:errorcluster, "Interface out"=w6485:refnum<class "Interface.lvclass">)  [unwired: 7 in]
                n2882 = call-dynamic "Read prev ExpTime.vi"("error in (no error)"=w6482, "Interface in"=w6485) -> ("error out"=w6479:errorcluster, "prev ExpTime"=w6480:dbl, "Interface out"=w6481:refnum<class "Interface.lvclass">)  [unwired: 7 in]
                n2883 = property on="Exptime ch4" class="DigNum (strict)"(error in=w6479, "Value"=w6480) -> (error out=w6478:errorcluster)  [unwired: 1 in, 1 out]
                n2884 = call "Write Exposure Time.vi"("error in (no error)"=w6478, "Exposure Time"=w6480, "Interface in"=w6481) -> ("error out"=w6477:errorcluster, "Interface out"=w6476:refnum<class "Interface.lvclass">)  [unwired: 7 in]
              }
            }
            n2885 = case shown="True" w6159 {
              tunnel: w6162 -> [w6488 w6499]
              tunnel: [w6488 w6489] -> w6165
              tunnel: w6160 -> [w6487 w6498]
              tunnel: [w6487 w6490] -> w6164
              frame False {
              }
              frame True {
                n2886 = call-dynamic "Write restoreExpTime.vi"("error in (no error)"=w6498, "restoreExpTime"=FALSE, "Interface in"=w6499) -> ("error out"=w6495:errorcluster, "Interface out"=w6496:refnum<class "Interface.lvclass">)  [unwired: 7 in]
                n2887 = call-dynamic "Read prev ExpTime.vi"("error in (no error)"=w6495, "Interface in"=w6496) -> ("error out"=w6492:errorcluster, "prev ExpTime"=w6493:dbl, "Interface out"=w6494:refnum<class "Interface.lvclass">)  [unwired: 7 in]
                n2888 = property on="Exptime ch3" class="DigNum (strict)"(error in=w6492, "Value"=w6493) -> (error out=w6491:errorcluster)  [unwired: 1 in, 1 out]
